vi "Oracle Popup.vi"(8 "error in":errorcluster) -> (0 "error out":errorcluster, 3 "SR array out":i32[](array[numeric]))   [LabVIEW 2018]
uses:
  <vilib>/Utility/miscctls.llb/LVPointTypeDef.ctl
panel:
  in  "Ok Button":bool
  in  "Copied Text":string
  in  "Close":bool
  # "In your Universal Work Queue in Oracle, right-click anywhere in the table and select \"Copy All Rows.\" Paste the copied information in the box below, then press \"OK\". This popup should only appear once, future refreshes will automatically pull from Oracle."
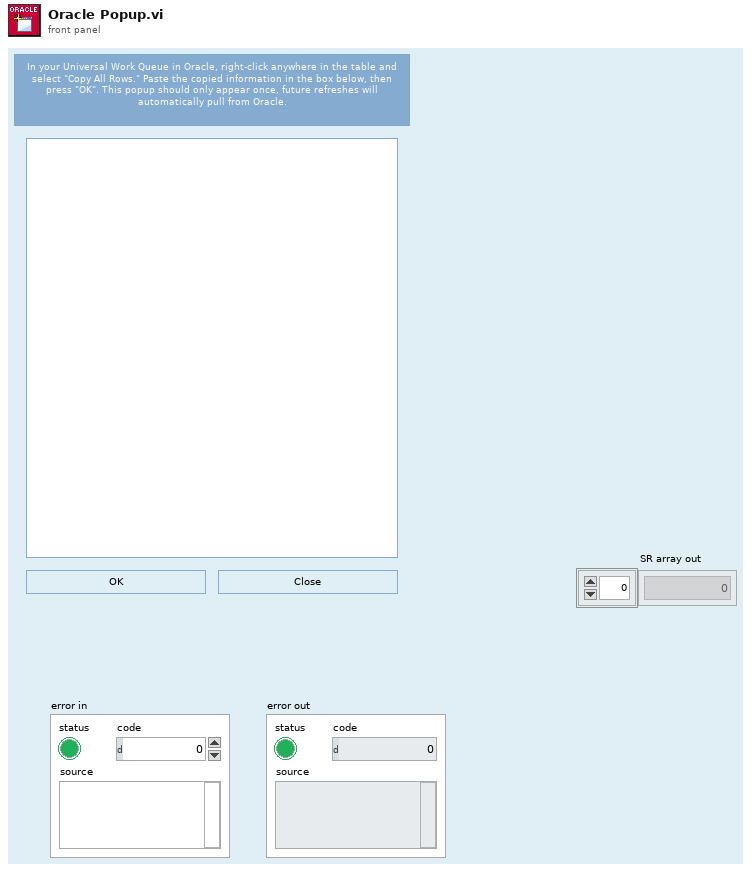
[diagram p1: front panel]
types:
  T1 = typedef "LVPointTypeDef.ctl" = cluster{"Horizontal":i16, "Vertical":i16}
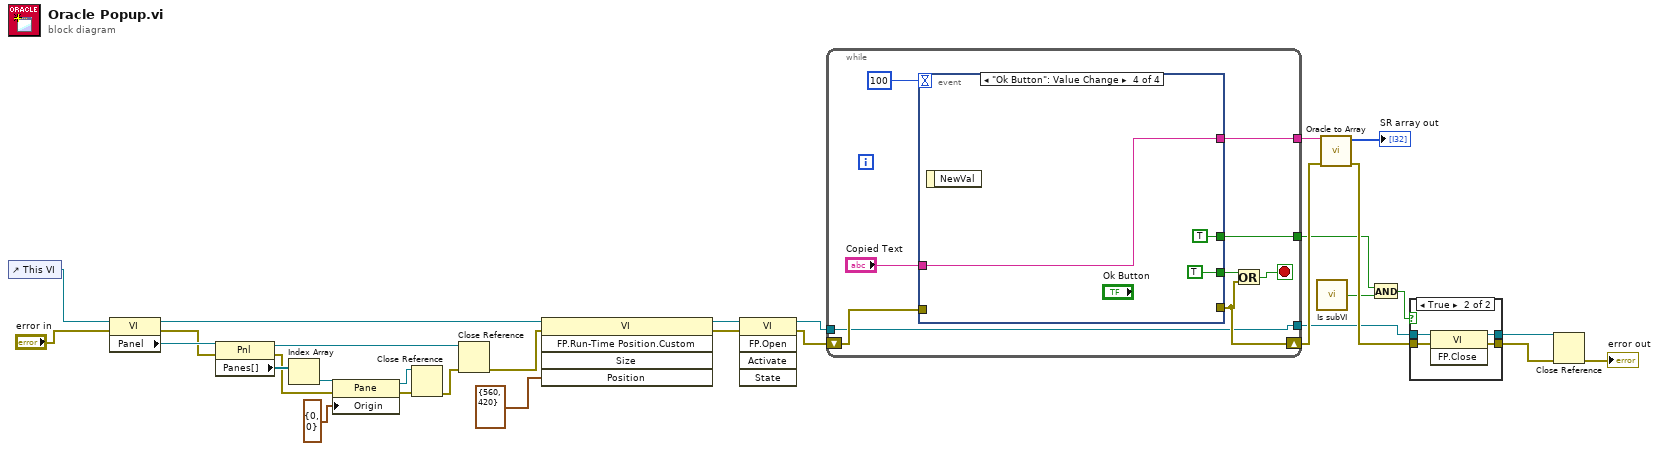
[diagram p0: block diagram]
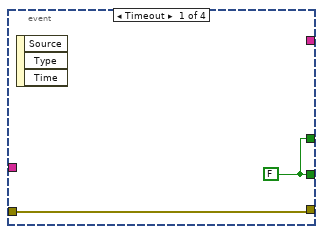
[diagram p2: hidden frame]
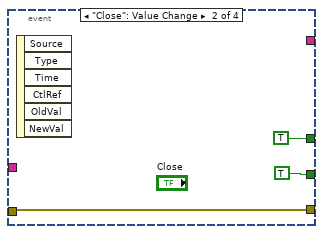
[diagram p3: hidden frame]
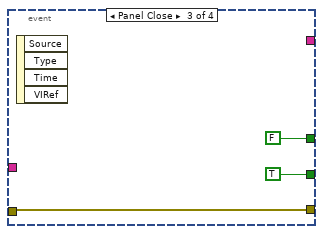
[diagram p4: hidden frame]
diagram:
  n1 = control-ref of="This VI"() -> (w10:refnum<vi>)
  n2 = property class="VI"(reference=w10, error in="error in") -> (reference out=w6:refnum<vi>, error out=w11:errorcluster, "Panel"=w12:refnum<vi>)
  n3 = property class="Pnl"(reference=w12, error in=w11) -> (reference out=w13:refnum<vi>, error out=w18:errorcluster, "Panes[]"=w20:refnum<vi>[])
  n4 = Index Array(array=w20) -> (element=w19:refnum<vi>)  [unwired: 1 in]
  n5 = property class="Pane"(reference=w19, error in=w18, "Origin"=T1 {"Horizontal"=0, "Vertical"=0}) -> (reference out=w16:refnum<vi>, error out=w15:errorcluster)
  n6 = Close Reference(reference=w16, error in (no error)=w15) -> (error out=w14:errorcluster)
  n7 = Close Reference(reference=w13, error in (no error)=w14) -> (error out=w5:errorcluster)
  n8 = invoke class="VI" method="FP.Run-Time Position.Custom"(reference=w6, error in=w5, "Position"=cluster{"Height":i16, "Width":i16} {"Height"=560, "Width"=420} ("Size")) -> (reference out=w8:refnum<vi>, error out=w7:errorcluster)  [unwired: 2 in, 3 out]
  n9 = invoke class="VI" method="FP.Open"(reference=w8, error in=w7) -> (reference out=w22:refnum<vi>, error out=w21:errorcluster)  [unwired: 3 in, 3 out]
  n10 = while {
    shift-right: [w34] -> w25
    shift-left: w21 -> [w37]
    tunnel: [w33] -> w2
    tunnel: [w32] -> w27
    tunnel: w22 -> [w31]
    tunnel: [w31] -> w23
    stop <- w35 stop-if-true
    n11 = event shown="[3] \"Ok Button\": Value Change" {
      selector: _ -> [_ _ _ _]
      dyn-events: _ -> [_ _ _ _]
      timeout: 100 -> [_ _ _ _]
      tunnel: [w40 TRUE ("Stop") TRUE ("Stop") TRUE ("Stop")] -> w36
      tunnel: "Copied Text" -> [_ _ _ w48]
      tunnel: w37 -> [w41 w43 w46 _]
      tunnel: [w41 w43 w46 _] -> w34
      tunnel: [w40 TRUE ("Stop") FALSE ("Stop") TRUE ("Stop")] -> w33
      tunnel: [_ _ _ w48] -> w32
      event Timeout {
        w40 = FALSE ("Stop")
        n12 = event-data() -> ()  [unwired: 1 in, 3 out]
      }
      event "Close": Value Change {
        n13 = event-data() -> ()  [unwired: 1 in, 6 out]
      }
      event Panel Close {
        n14 = event-data() -> ()  [unwired: 1 in, 4 out]
      }
      event "Ok Button": Value Change {
        n15 = event-data() -> ()  [unwired: 1 in, 1 out]
      }
    }
    n16 = Or(x=w36, y=w34) -> (x .or. y?=w35:bool)
  }
  n17 = call "Is subVI.vi"() -> ("Is subVI?"=w1:bool)  [unwired: 1 in]
  n18 = call "Oracle to Array.vi"("error in"=w25, "string in"=w27) -> ("error out"=w24:errorcluster, "SR number array out"=→"SR array out":i32[])  [unwired: 7 in, 1 out]
  n19 = And(x=w2, y=w1) -> (x .and. y?=w3:bool)
  n20 = case shown="True" w3 {
    tunnel: w23 -> [w52 w56]
    tunnel: w24 -> [w51 w55]
    tunnel: [w52 w54] -> w30
    tunnel: [w51 w53] -> w29
    frame False {
    }
    frame True {
      n21 = invoke class="VI" method="FP.Close"(reference=w56, error in=w55) -> (reference out=w54:refnum<vi>, error out=w53:errorcluster)  [unwired: 1 in, 1 out]
    }
  }
  n22 = Close Reference(reference=w30, error in (no error)=w29) -> (error out=→"error out":errorcluster)
